vi "All Laser Com.vi"(11 "Network":T1) -> ()   [LabVIEW 2023]
uses:
  TypeDefs/Network_config.ctl
  TypeDefs/laser_cabinet_status.ctl
  Globals/Globals.vi
panel:
  out "Data size N2":u32
  out "Data size S2":u32
  out "Data size N1":u32
  out "Data size S1":u32
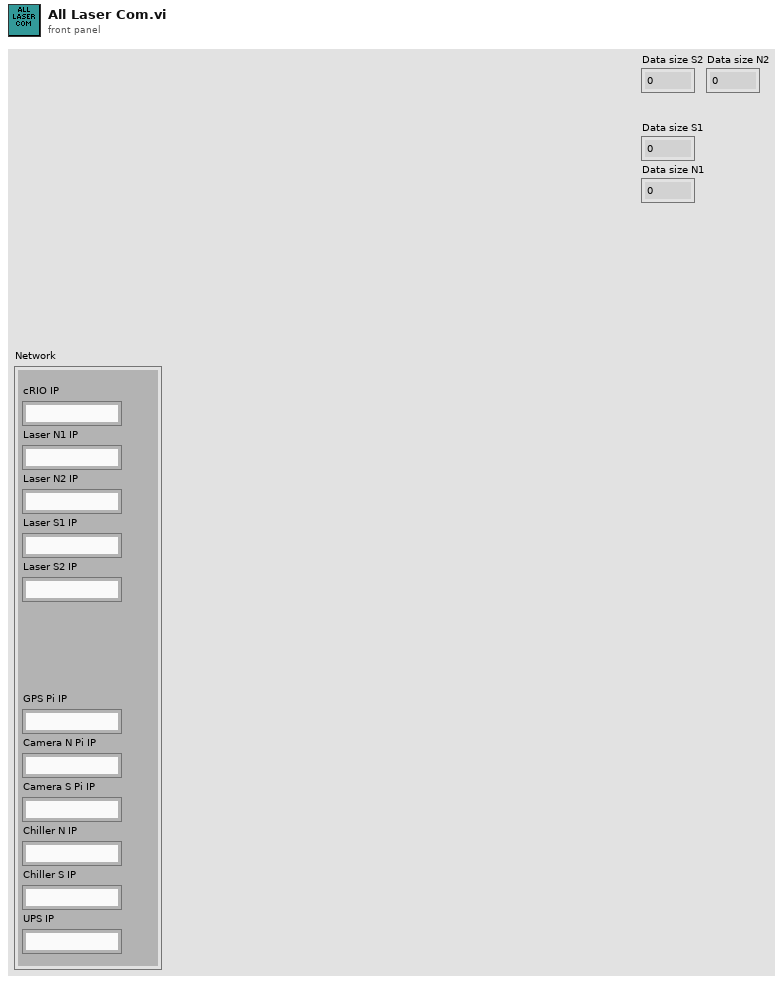
[diagram p1: front panel]
types:
  T1 = typedef "Network_config.ctl" = cluster{"cRIO IP":string, "Laser N1 IP":string, "Laser N2 IP":string, "Laser S1 IP":string, "Laser S2 IP":string, "GPS Pi IP":string, "Camera N Pi IP":string, "Camera S Pi IP":string, "Chiller N IP":string, "Chiller S IP":string, "UPS IP":string}
  T2 = typedef "laser_cabinet_status.ctl" = cluster{"Version":u16, "Installed Status":u32, "Set Mode Index":u16, "Set Frequency (kHz)":sgl, "Average Power (W)":sgl, "Set Power (%)":sgl, "Main Status":u32, "Alarms":u32, "System Alarms":u32, "Extended Alarms":u32, "Warnings":u32, "Status":u32, "Extended Status":u32, "Reserved1":u16, "Measured Frequency (kHz)":sgl, "Pulse Duration (ns)":u32, "Measured Power (W)":sgl, "Pulse Energy (mJ)":sgl, "Peak Power (kW)":sgl, "Analog power control (mV)":sgl, "Back Reflection (mV)":sgl, "PS mean (C)":sgl, "PS max (C)":sgl, "PS min (C)":sgl, "Dew Point (C)":sgl, "Remote Controller Temperature (C)":sgl, "Isolator Temperature (C)":sgl, "MO mean (C)":sgl, "MO max (C)":sgl, "MO min (C)":sgl, "PA mean (C)":sgl, "PA max (C)":sgl, "PA min (C)":sgl, "BS mean (C)":sgl, "BS max (C)":sgl, "BS min (C)":sgl, "Humidity (%)":sgl}
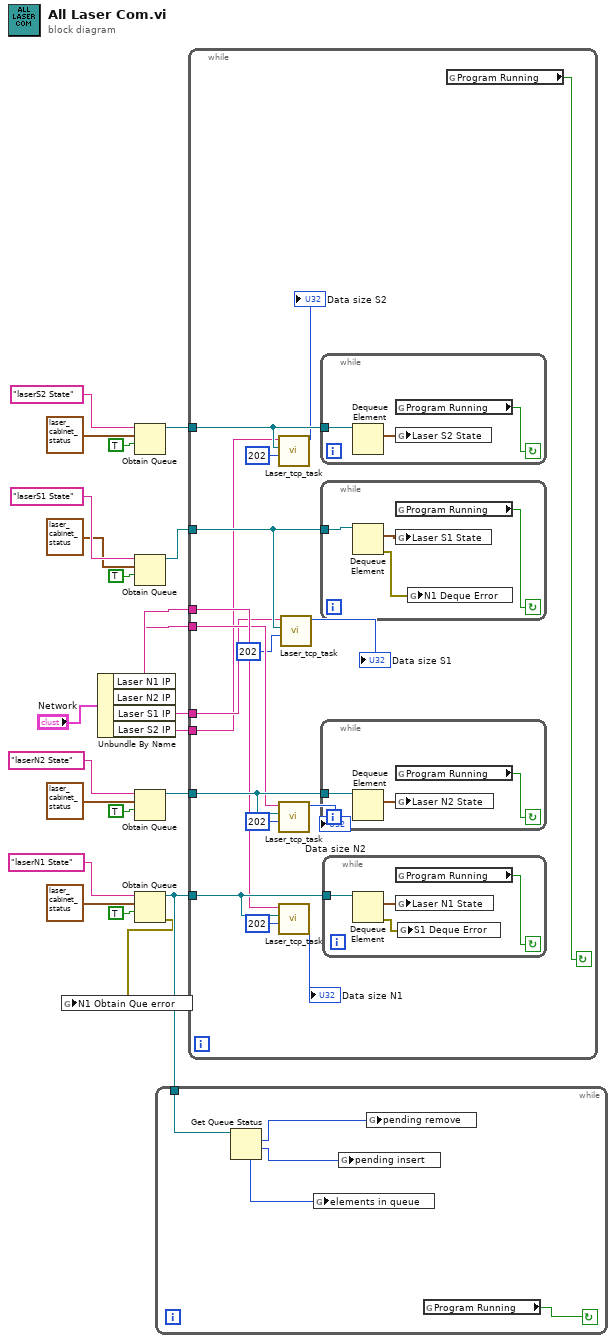
[diagram p0: block diagram]
diagram:
  n1 = Unbundle By Name("Network") -> ("Laser N1 IP"=w6:string, "Laser N2 IP"=w5:string, "Laser S1 IP"=w4:string, "Laser S2 IP"=w3:string)
  n2 = Obtain Queue(name (unnamed)="laserS2 State", element data type=T2 {"Version"=1, "Installed Status"=0, "Set Mode Index"=0, "Set Frequency (kHz)"=0.0, "Average Power (W)"=0.0, "Set Power (%)"=0.0, "Main Status"=1, "Alarms"=32, "System Alarms"=0, "Extended Alarms"=0, "Warnings"=0, "Status"=0, "Extended Status"=0, "Reserved1"=0, "Measured Frequency (kHz)"=0.0, "Pulse Duration (ns)"=0, "Measured Power (W)"=0.0, "Pulse Energy (mJ)"=0.0, "Peak Power (kW)"=0.0, "Analog power control (mV)"=0.0, "Back Reflection (mV)"=0.0, "PS mean (C)"=0.0, "PS max (C)"=0.0, "PS min (C)"=0.0, "Dew Point (C)"=0.0, "Remote Controller Temperature (C)"=0.0, "Isolator Temperature (C)"=0.0, "MO mean (C)"=0.0, "MO max (C)"=0.0, "MO min (C)"=0.0, "PA mean (C)"=0.0, "PA max (C)"=0.0, "PA min (C)"=0.0, "BS mean (C)"=0.0, "BS max (C)"=0.0, "BS min (C)"=0.0, "Humidity (%)"=0.0} ("output cluster"), create if not found? (T)=TRUE) -> (queue out=w12:refnum<queue>)  [unwired: 2 in, 2 out]
  n3 = Obtain Queue(name (unnamed)="laserS1 State", element data type=T2 {"Version"=1, "Installed Status"=0, "Set Mode Index"=0, "Set Frequency (kHz)"=0.0, "Average Power (W)"=0.0, "Set Power (%)"=0.0, "Main Status"=1, "Alarms"=32, "System Alarms"=0, "Extended Alarms"=0, "Warnings"=0, "Status"=0, "Extended Status"=0, "Reserved1"=0, "Measured Frequency (kHz)"=0.0, "Pulse Duration (ns)"=0, "Measured Power (W)"=0.0, "Pulse Energy (mJ)"=0.0, "Peak Power (kW)"=0.0, "Analog power control (mV)"=0.0, "Back Reflection (mV)"=0.0, "PS mean (C)"=0.0, "PS max (C)"=0.0, "PS min (C)"=0.0, "Dew Point (C)"=0.0, "Remote Controller Temperature (C)"=0.0, "Isolator Temperature (C)"=0.0, "MO mean (C)"=0.0, "MO max (C)"=0.0, "MO min (C)"=0.0, "PA mean (C)"=0.0, "PA max (C)"=0.0, "PA min (C)"=0.0, "BS mean (C)"=0.0, "BS max (C)"=0.0, "BS min (C)"=0.0, "Humidity (%)"=0.0} ("output cluster"), create if not found? (T)=TRUE) -> (queue out=w11:refnum<queue>)  [unwired: 2 in, 2 out]
  n4 = Obtain Queue(name (unnamed)="laserN2 State", element data type=T2 {"Version"=1, "Installed Status"=0, "Set Mode Index"=0, "Set Frequency (kHz)"=0.0, "Average Power (W)"=0.0, "Set Power (%)"=0.0, "Main Status"=1, "Alarms"=32, "System Alarms"=0, "Extended Alarms"=0, "Warnings"=0, "Status"=0, "Extended Status"=0, "Reserved1"=0, "Measured Frequency (kHz)"=0.0, "Pulse Duration (ns)"=0, "Measured Power (W)"=0.0, "Pulse Energy (mJ)"=0.0, "Peak Power (kW)"=0.0, "Analog power control (mV)"=0.0, "Back Reflection (mV)"=0.0, "PS mean (C)"=0.0, "PS max (C)"=0.0, "PS min (C)"=0.0, "Dew Point (C)"=0.0, "Remote Controller Temperature (C)"=0.0, "Isolator Temperature (C)"=0.0, "MO mean (C)"=0.0, "MO max (C)"=0.0, "MO min (C)"=0.0, "PA mean (C)"=0.0, "PA max (C)"=0.0, "PA min (C)"=0.0, "BS mean (C)"=0.0, "BS max (C)"=0.0, "BS min (C)"=0.0, "Humidity (%)"=0.0} ("output cluster"), create if not found? (T)=TRUE) -> (queue out=w19:refnum<queue>)  [unwired: 2 in, 2 out]
  n5 = Obtain Queue(name (unnamed)="laserN1 State", element data type=T2 {"Version"=1, "Installed Status"=0, "Set Mode Index"=0, "Set Frequency (kHz)"=0.0, "Average Power (W)"=0.0, "Set Power (%)"=0.0, "Main Status"=1, "Alarms"=32, "System Alarms"=0, "Extended Alarms"=0, "Warnings"=0, "Status"=0, "Extended Status"=0, "Reserved1"=0, "Measured Frequency (kHz)"=0.0, "Pulse Duration (ns)"=0, "Measured Power (W)"=0.0, "Pulse Energy (mJ)"=0.0, "Peak Power (kW)"=0.0, "Analog power control (mV)"=0.0, "Back Reflection (mV)"=0.0, "PS mean (C)"=0.0, "PS max (C)"=0.0, "PS min (C)"=0.0, "Dew Point (C)"=0.0, "Remote Controller Temperature (C)"=0.0, "Isolator Temperature (C)"=0.0, "MO mean (C)"=0.0, "MO max (C)"=0.0, "MO min (C)"=0.0, "PA mean (C)"=0.0, "PA max (C)"=0.0, "PA min (C)"=0.0, "BS mean (C)"=0.0, "BS max (C)"=0.0, "BS min (C)"=0.0, "Humidity (%)"=0.0} ("output cluster"), create if not found? (T)=TRUE) -> (queue out=w2:refnum<queue>, error out=w1:errorcluster)  [unwired: 2 in, 1 out]
  n6 = global write "Globals.vi" "N1 Obtain Que error"(w1) -> ()
  n7 = while {
    tunnel: w2 -> [w27]
    stop <- w26 continue-if-true
    n8 = Get Queue Status(queue=w27) -> (# pending remove=w25:i32, # pending insert=w24:i32, # elements in queue=w23:i32)  [unwired: 2 in, 5 out]
    n9 = global write "Globals.vi" "elements in queue"(w23) -> ()
    n10 = global write "Globals.vi" "pending insert"(w24) -> ()
    n11 = global write "Globals.vi" "pending remove"(w25) -> ()
    n12 = global read "Globals.vi" "Program Running"() -> (w26:bool)
  }
  n13 = while {
    tunnel: w2 -> [w44]
    tunnel: w19 -> [w43]
    tunnel: w11 -> [w41]
    tunnel: w12 -> [w42]
    tunnel: w6 -> [w40]
    tunnel: w5 -> [w39]
    tunnel: w4 -> [w38]
    tunnel: w3 -> [w37]
    stop <- w36 continue-if-true
    n14 = call "Laser_tcp_task.vi"("bytes to read"=202, "queue out"=w42, "address"=w37) -> ("Data size"=→"Data size S2":u32)  [unwired: 8 in]
    n15 = call "Laser_tcp_task.vi"("bytes to read"=202, "queue out"=w43, "address"=w39) -> ("Data size"=→"Data size N2":u32)  [unwired: 8 in]
    n16 = call "Laser_tcp_task.vi"("bytes to read"=202, "queue out"=w44, "address"=w40) -> ("Data size"=→"Data size N1":u32)  [unwired: 8 in]
    n17 = call "Laser_tcp_task.vi"("bytes to read"=202, "queue out"=w41, "address"=w38) -> ("Data size"=→"Data size S1":u32)  [unwired: 8 in]
    n18 = while {
      tunnel: w42 -> [w50]
      stop <- w49 continue-if-true
      n19 = Dequeue Element(queue=w50) -> (element=w48:T2)  [unwired: 2 in, 3 out]
      n20 = global read "Globals.vi" "Program Running"() -> (w49:bool)
      n21 = global write "Globals.vi" "Laser S2 State"(w48) -> ()
    }
    n22 = while {
      tunnel: w41 -> [w58]
      stop <- w57 continue-if-true
      n23 = Dequeue Element(queue=w58) -> (element=w56:T2, error out=w55:errorcluster)  [unwired: 2 in, 2 out]
      n24 = global read "Globals.vi" "Program Running"() -> (w57:bool)
      n25 = global write "Globals.vi" "Laser S1 State"(w56) -> ()
      n26 = global write "Globals.vi" "N1 Deque Error"(w55) -> ()
    }
    n27 = while {
      tunnel: w43 -> [w47]
      stop <- w46 continue-if-true
      n28 = Dequeue Element(queue=w47) -> (element=w45:T2)  [unwired: 2 in, 3 out]
      n29 = global read "Globals.vi" "Program Running"() -> (w46:bool)
      n30 = global write "Globals.vi" "Laser N2 State"(w45) -> ()
    }
    n31 = while {
      tunnel: w44 -> [w54]
      stop <- w53 continue-if-true
      n32 = Dequeue Element(queue=w54) -> (element=w52:T2, error out=w51:errorcluster)  [unwired: 2 in, 2 out]
      n33 = global read "Globals.vi" "Program Running"() -> (w53:bool)
      n34 = global write "Globals.vi" "Laser N1 State"(w52) -> ()
      n35 = global write "Globals.vi" "S1 Deque Error"(w51) -> ()
    }
    n36 = global read "Globals.vi" "Program Running"() -> (w36:bool)
  }
